vi "User32dllAPI.GetDisplaysOld.vi"() -> (0 "#displays":i32, 1 "width":i32, 2 "total width":i32, 3 "offset":i32, 4 "height":i32)   [LabVIEW 2015]
uses:
  user32.dll
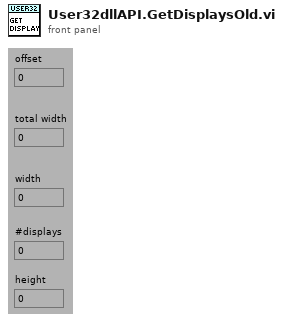
[diagram p1: front panel]
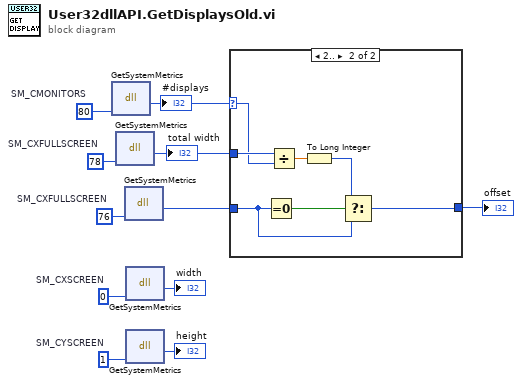
[diagram p0: block diagram]
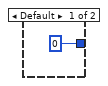
[diagram p2: hidden frame]
diagram:
  w1 = 1  # SM_CYSCREEN
  w4 = 0  # SM_CXSCREEN
  w8 = 76  # SM_CXFULLSCREEN
  w9 = 78  # SM_CXFULLSCREEN
  w11 = 80  # SM_CMONITORS
  n1 = dll-call lib="USER32.DLL" fn="GetSystemMetrics"("parameter"=w11) -> ("screenWidth"=w10:i32)  [unwired: 4 in, 2 out]
  "#displays" <- w10
  n2 = dll-call lib="USER32.DLL" fn="GetSystemMetrics"("parameter"=w9) -> ("screenHeight"=w7:i32)  [unwired: 4 in, 2 out]
  "total width" <- w7
  n3 = dll-call lib="USER32.DLL" fn="GetSystemMetrics"("parameter"=w8) -> ("screenHeight"=w6:i32)  [unwired: 4 in, 2 out]
  n4 = dll-call lib="USER32.DLL" fn="GetSystemMetrics"("parameter"=w4) -> ("screenWidth"=→"width":i32)  [unwired: 4 in, 2 out]
  n5 = dll-call lib="USER32.DLL" fn="GetSystemMetrics"("parameter"=w1) -> ("screenWidth"=→"height":i32)  [unwired: 4 in, 2 out]
  n6 = case shown="2.." w10 {
    selector: w10 -> [_ w13]
    tunnel: w7 -> [_ w19]
    tunnel: w6 -> [_ w15]
    tunnel: [0 ("screenHeight") w14] -> w5
    frame Default {
    }
    frame 2.. {
      n7 = Equal To 0?(x=w15) -> (x = 0?=w18:bool)
      n8 = Divide(x=w19, y=w13) -> (x/y=w17:dbl)
      n9 = To Long Integer(number=w17) -> (32bit integer=w16:i32)
      n10 = Select(t=w16, s=w18, f=w15) -> (s? t:f=w14:i32)
    }
  }
  "offset" <- w5
